vi "LJT4_V2T.vi"(8 "CJC (K)":dbl, 11 "voltage_array":dbl[](array[numeric])) -> (0 "array_mV":dbl[](array[numeric]), 1 "array_T_F":dbl[](array[numeric]), 2 "array_T_C":dbl[](array[numeric]), 3 "array_T_K":dbl[](array[numeric]))   [LabVIEW 2019]
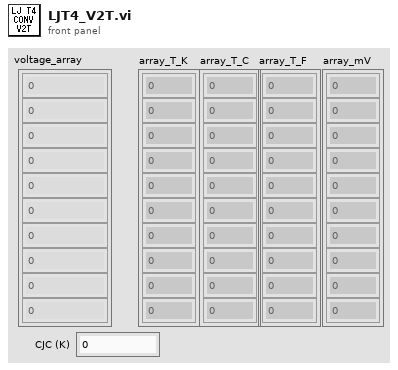
[diagram p1: front panel]
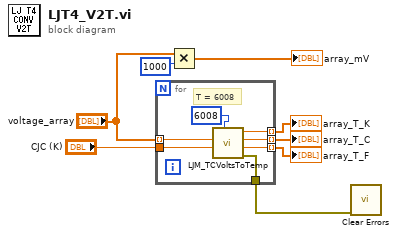
[diagram p0: block diagram]
diagram:
  n1 = for {
    tunnel: "voltage_array" -> [w11] mode=indexing
    tunnel: [w12] -> w8 mode=indexing
    tunnel: [w14] -> w6 mode=indexing
    tunnel: [w13] -> w7 mode=indexing
    tunnel: "CJC (K)" -> [w10]
    tunnel: [w9] -> w1
    # "T = 6008"
    n2 = call "LJM_TCVoltsToTemp.vi"("TCType"=6008, "CJTempK"=w10, "TCVolts"=w11) -> ("error out"=w9:errorcluster, "TCTempF"=w12:dbl, "TCTempC"=w13:dbl, "TCTempK"=w14:dbl)  [unwired: 5 in]
  }
  "array_T_F" <- w8
  "array_T_C" <- w7
  "array_T_K" <- w6
  n3 = Multiply(x="voltage_array", y=1000) -> (x*y=→"array_mV":dbl[])
  n4 = call <vilib>:"Clear Errors.vi"("error in (no error)"=w1) -> ()  [unwired: 5 in, 2 out]
